vi "StartPull.vi"(2 "error in":errorcluster, 3 "Master Axis":i32, 4 "VISA resource name":refnum<visa-resource-name>) -> (0 "error out":errorcluster, 1 "VISA resource name out":refnum<visa-resource-name>)   [LabVIEW 2009]
uses:
  <instrlib>/Newport ESP301/Newport ESP301.lvlib
panel:
  in  "Slave Axis":i32
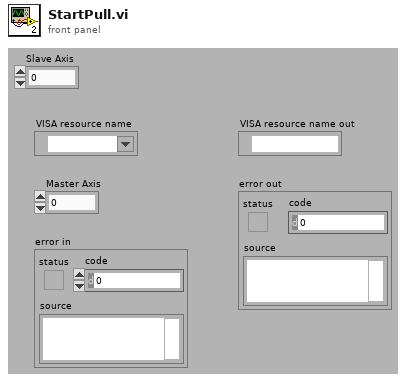
[diagram p1: front panel]
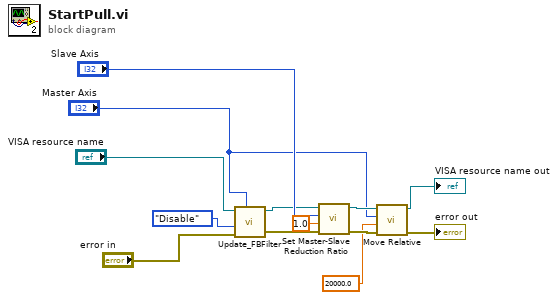
[diagram p0: block diagram]
diagram:
  n1 = call "Update_FBFilter.vi"("Axis"="Master Axis", "error in (no error)"="error in", "Disable?"=enum16{"Disable", "Set"}."Disable", "VISA resource name"="VISA resource name") -> ("error out"=w8:errorcluster, "VISA resource name out"=w9:refnum<visa-resource-name>)  [unwired: 6 in]
  n2 = call <instrlib>:"Set Master-Slave Reduction Ratio.vi"("error in (no error)"=w8, "Reduction Ratio (0)"=1.0, "Axis (1)"="Slave Axis", "VISA resource name"=w9) -> ("error out"=w4:errorcluster, "VISA resource name out"=w7:refnum<visa-resource-name>)  [unwired: 2 in]
  n3 = call <instrlib>:"Move Relative.vi"("error in (no error)"=w4, "Position (0 units)"=20000.0, "Axis (1)"="Master Axis", "VISA resource name"=w7) -> ("error out"=→"error out":errorcluster, "VISA resource name out"=→"VISA resource name out":refnum<visa-resource-name>)  [unwired: 2 in]
